vi "gfitsio-read-column-u8-1d.vi"(6 "row":i32, 7 "column":string, 8 "error in (no error)":errorcluster, 11 "gfits refnum":T1) -> (0 "error out":errorcluster, 2 "data":u8[](array[numeric]), 3 "dup gfits refnum":T1)   [LabVIEW 2011, in "gfitsio.lvlib"]
doc: "Read elements from an ASCII or binary table column."
uses:
  gfitsio.lvlib
  gfitsio-refnum.ctl
  cfitsio-hdutypes.ctl
  gfitsio.dll
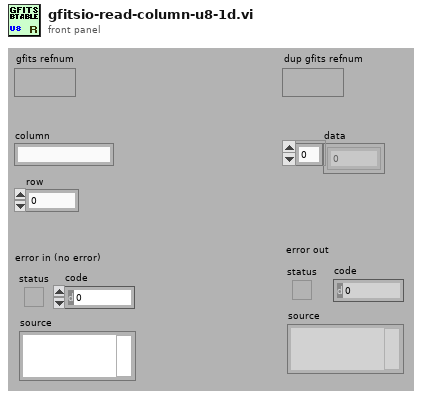
[diagram p1: front panel]
types:
  T1 = typedef "gfitsio.lvlib/gfitsio-refnum.ctl" = refnum<k1>
  T2 = typedef "gfitsio.lvlib/cfitsio-hdutypes.ctl" = i32
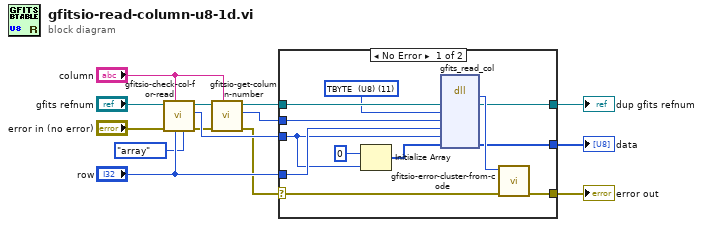
[diagram p0: block diagram]
diagram:
  n1 = call "gfitsio-check-col-for-read.vi"("expected dimensionality"=enum16{"scalar", "array"}."array", "row"="row", "column"="column", "error in (no error)"="error in (no error)", "gfits refnum"="gfits refnum") -> ("error out"=w5:errorcluster, "nelements"=w10:i32, "dup gfits refnum"=w6:T1)  [unwired: 4 in]
  n2 = call "gfitsio-get-column-number.vi"("column"="column", "error in (no error)"=w5, "gfits refnum"=w6) -> ("error out"=w4:errorcluster, "colnum"=w1:i32, "dup gfits refnum"=w3:T1)  [unwired: 6 in]
  n3 = case shown="No Error" w4 {
    selector: w4 -> [w26 w28]
    tunnel: [w25 w28] -> w13
    tunnel: w3 -> [w22 w27]
    tunnel: [w23 w27] -> w9
    tunnel: "row" -> [w20 _]
    tunnel: [w21 _] -> w14
    tunnel: w10 -> [w19 _]
    tunnel: w1 -> [w16 _]
    frame No Error {
      w15 = T2 11 items=["TBIT"=1, "TBYTE  (U8)"=11, "TSBYTE  (I8)"=12, "TLOGICAL"=14, "TSTRING"=16, "TUSHORT  (U16)"=20, "TSHORT  (I16)"=21, "TUINT"=31, "TULONG  (U32)"=40, "TLONG  (I32)"=41, "TFLOAT  (SGL)"=42, "TLONGLONG  (I64)"=81, "TDOUBLE"=82, "TCOMPLEX  (CSG)"=83, "TDOUBLECOMPLEX  (CDB)"=163] ("cfitsio datatype")
      n4 = Initialize Array(u8 0 ("element"), w19) -> (w17:u8[])
      n5 = dll-call lib="C:/BonOMM/BonOMM-SAOMM/SubVIs/gfitsio/gfitsio.dll" fn="gfits_read_col"("dup gfits refnum"=w22, "datatype"=w15, "colnum"=w16, "row"=w20, "nelements"=w19, "data"=w17) -> (w24:i32, "dup gfits refnum"=w23:T1, "data"=w21:u8[])  [unwired: 7 in, 2 out]
      n6 = call "gfitsio-error-cluster-from-code.vi"("error in (no error)"=w26, "error code"=w24) -> ("error out"=w25:errorcluster)  [unwired: 9 in]
    }
    frame Error {
    }
  }
  "error out" <- w13
  "dup gfits refnum" <- w9
  "data" <- w14
